vi "Start.vi"(8 "error in (no error)":errorcluster, 11 "HAL GOOP4:Series Base in":refnum<class "Series Base.lvclass">) -> (0 "error out":errorcluster, 3 "HAL GOOP4:Series Base out":refnum<class "Series Base.lvclass">)   [LabVIEW 2023, in "HAL GOOP4.lvlib" / "Series Base.lvclass"]
uses:
  Series Base.lvclass
  Series Base.lvclass/Series Base.ctl
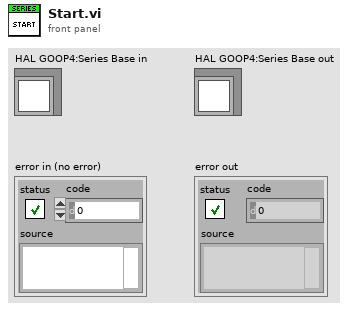
[diagram p1: front panel]
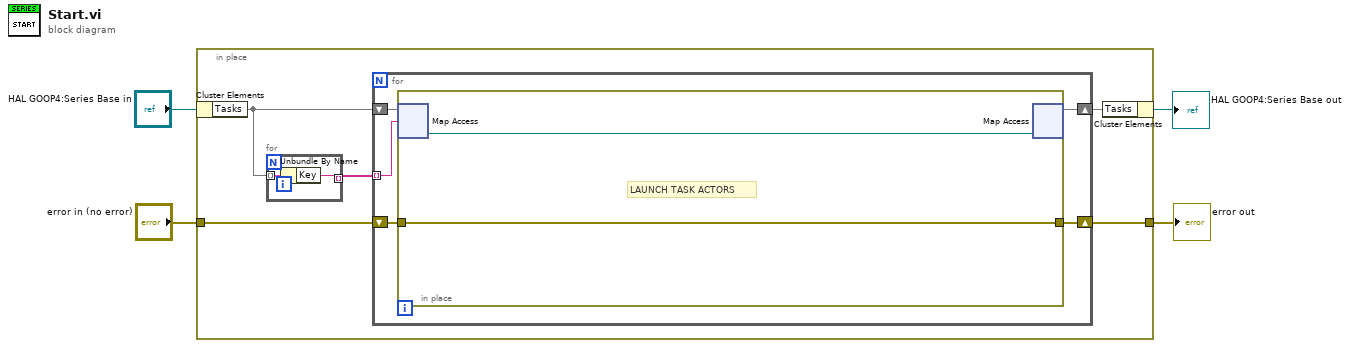
[diagram p0: block diagram]
diagram:
  n1 = in-place {
    in-place-border: "error in (no error)" -> [w5]
    in-place-border: [w9] -> w2
    n2 = in-place-cluster #1("HAL GOOP4:Series Base in") -> ("Tasks"=w7:map{string, refnum<class "Task Base.lvclass">})
    n3 = for {
      tunnel: [w18] -> w8 mode=indexing
      tunnel: w7 -> [w17] mode=indexing
      n4 = Unbundle By Name(w17) -> ("Key"=w18:string)
    }
    n5 = for {
      tunnel: w8 -> [w12] mode=indexing
      shift-right: [w11] -> w6
      shift-left: w7 -> [w13]
      shift-right: [w14] -> w9
      shift-left: w5 -> [w10]
      n6 = in-place {
        in-place-border: [w15] -> w14
        in-place-border: w10 -> [w15]
        # "LAUNCH TASK ACTORS"
        n7 = in-place-map #2(w13, w12) -> (w16:refnum<class "Task Base.lvclass">)  [unwired: 1 in, 1 out]
        n8 = in-place-map #2(w16) -> (w11:map{string, refnum<class "Task Base.lvclass">})  [unwired: 1 in, 2 out]
      }
    }
    n9 = in-place-cluster #1("Tasks"=w6) -> (→"HAL GOOP4:Series Base out":refnum<class "Series Base.lvclass">)
  }
  "error out" <- w2
